vi "sub_isCellEmpty.vi"(9 "selection index":i32, 11 "control references":refnum<vi>[](array[refnum])) -> (2 "empty?":bool)   [LabVIEW 2018]
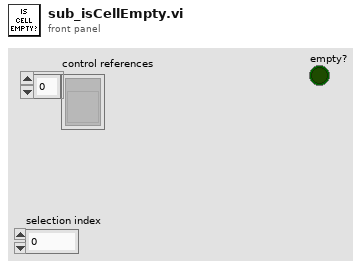
[diagram p1: front panel]
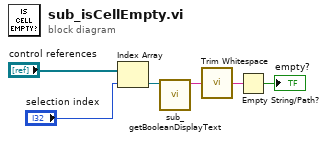
[diagram p0: block diagram]
diagram:
  n1 = Index Array(array="control references", index="selection index") -> (element=w2:refnum<vi>)
  n2 = call "sub_getBooleanDisplayText.vi"(11:w2) -> ("True Label"=w1:string)  [unwired: 10 in]
  n3 = call <vilib>:"Trim Whitespace.vi"("string"=w1) -> ("trimmed string"=w4:string)  [unwired: 1 in]
  n4 = Empty String/Path?(string/path=w4) -> (empty?=→"empty?":bool)
